vi "APDM Get Gyro Data.vi"(5 "Sim Gyro Cluster":T1, 8 "Gyro Data":T3={"Time"=0.0, "Normalization Time"=640.0, "Sampling Rate"=0.0, "Left Gyro Data"={"Time"=0.0, "Gyro Array Data"=[], "Gyro Negation"=[], "Gyro Data"={"Gyro X"=0.0, "Gyro Y"=0.0, "Gyro Z"=0.0}, "Gyro Latency"=0.0, "Normalization Time"=0.0, "Sampling Rate"=0.0}, "Right Gyro Data"={"Time"=0.0, "Gyro Array Data"=[], "Gyro Negation"=[], "Gyro Data"={"Gyro X"=0.0, "Gyro Y"=0.0, "Gyro Z"=0.0}, "Gyro Latency"=0.0, "Normalization Time"=0.0, "Sampling Rate"=0.0}}, 9 "APDM Context":T6={"APDM Context ID"=0, "Gyro Mode"="", "Log Data"=FALSE, "Log File"=refnum, "Gyro Record Log"=refnum, "Gyro CMD Log"=refnum, "L Opal SN"=0, "R Opal SN"=0, "Access Point ID"=0, "Left Gyro Sim Data"=path "C:/Users/jfalesi/Desktop/CP FES Walking Code/Original/Ahad Vi/CP Code/Offline data/TD_7_Raw_R.txt", "Right Gyro Sim Data"=path "C:/Users/jfalesi/Desktop/CP FES Walking Code/Original/Ahad Vi/CP Code/Offline data/TD_7_Raw_R.txt", "Sampling Rate"=0.0, "Gyro Sim Time Array"=[], "Missed Gyro Count"=0.0}) -> (1 "Cmd Log String":string, 2 "Gyro Data":T3={"Time"=0.0, "Normalization Time"=640.0, "Sampling Rate"=0.0, "Left Gyro Data"={"Time"=0.0, "Gyro Array Data"=[], "Gyro Negation"=[], "Gyro Data"={"Gyro X"=0.0, "Gyro Y"=0.0, "Gyro Z"=0.0}, "Gyro Latency"=0.0, "Normalization Time"=0.0, "Sampling Rate"=0.0}, "Right Gyro Data"={"Time"=0.0, "Gyro Array Data"=[], "Gyro Negation"=[], "Gyro Data"={"Gyro X"=0.0, "Gyro Y"=0.0, "Gyro Z"=0.0}, "Gyro Latency"=0.0, "Normalization Time"=0.0, "Sampling Rate"=0.0}}, 3 "APDM Context Out out":T6={"APDM Context ID"=0, "Gyro Mode"="", "Log Data"=FALSE, "Log File"=refnum, "Gyro Record Log"=refnum, "Gyro CMD Log"=refnum, "L Opal SN"=0, "R Opal SN"=0, "Access Point ID"=0, "Left Gyro Sim Data"=path "C:/Users/jfalesi/Desktop/CP FES Walking Code/Original/Ahad Vi/CP Code/Offline data/TD_7_Raw_R.txt", "Right Gyro Sim Data"=path "C:/Users/jfalesi/Desktop/CP FES Walking Code/Original/Ahad Vi/CP Code/Offline data/TD_7_Raw_R.txt", "Sampling Rate"=0.0, "Gyro Sim Time Array"=[], "Missed Gyro Count"=0.0}, 4 "Data Log Item":T2)   [LabVIEW 2019]
uses:
  Controls/APDM Context Cluster.ctl
  Controls/Gyro Data.ctl
  Controls/Gyro Side Data.ctl
  Controls/Gyro Negation.ctl
  Controls/Gyro Data Log Item.ctl
  Archive/CP_FES_Walking_w_stim_on_off.llb/Left_Right_Control.ctl
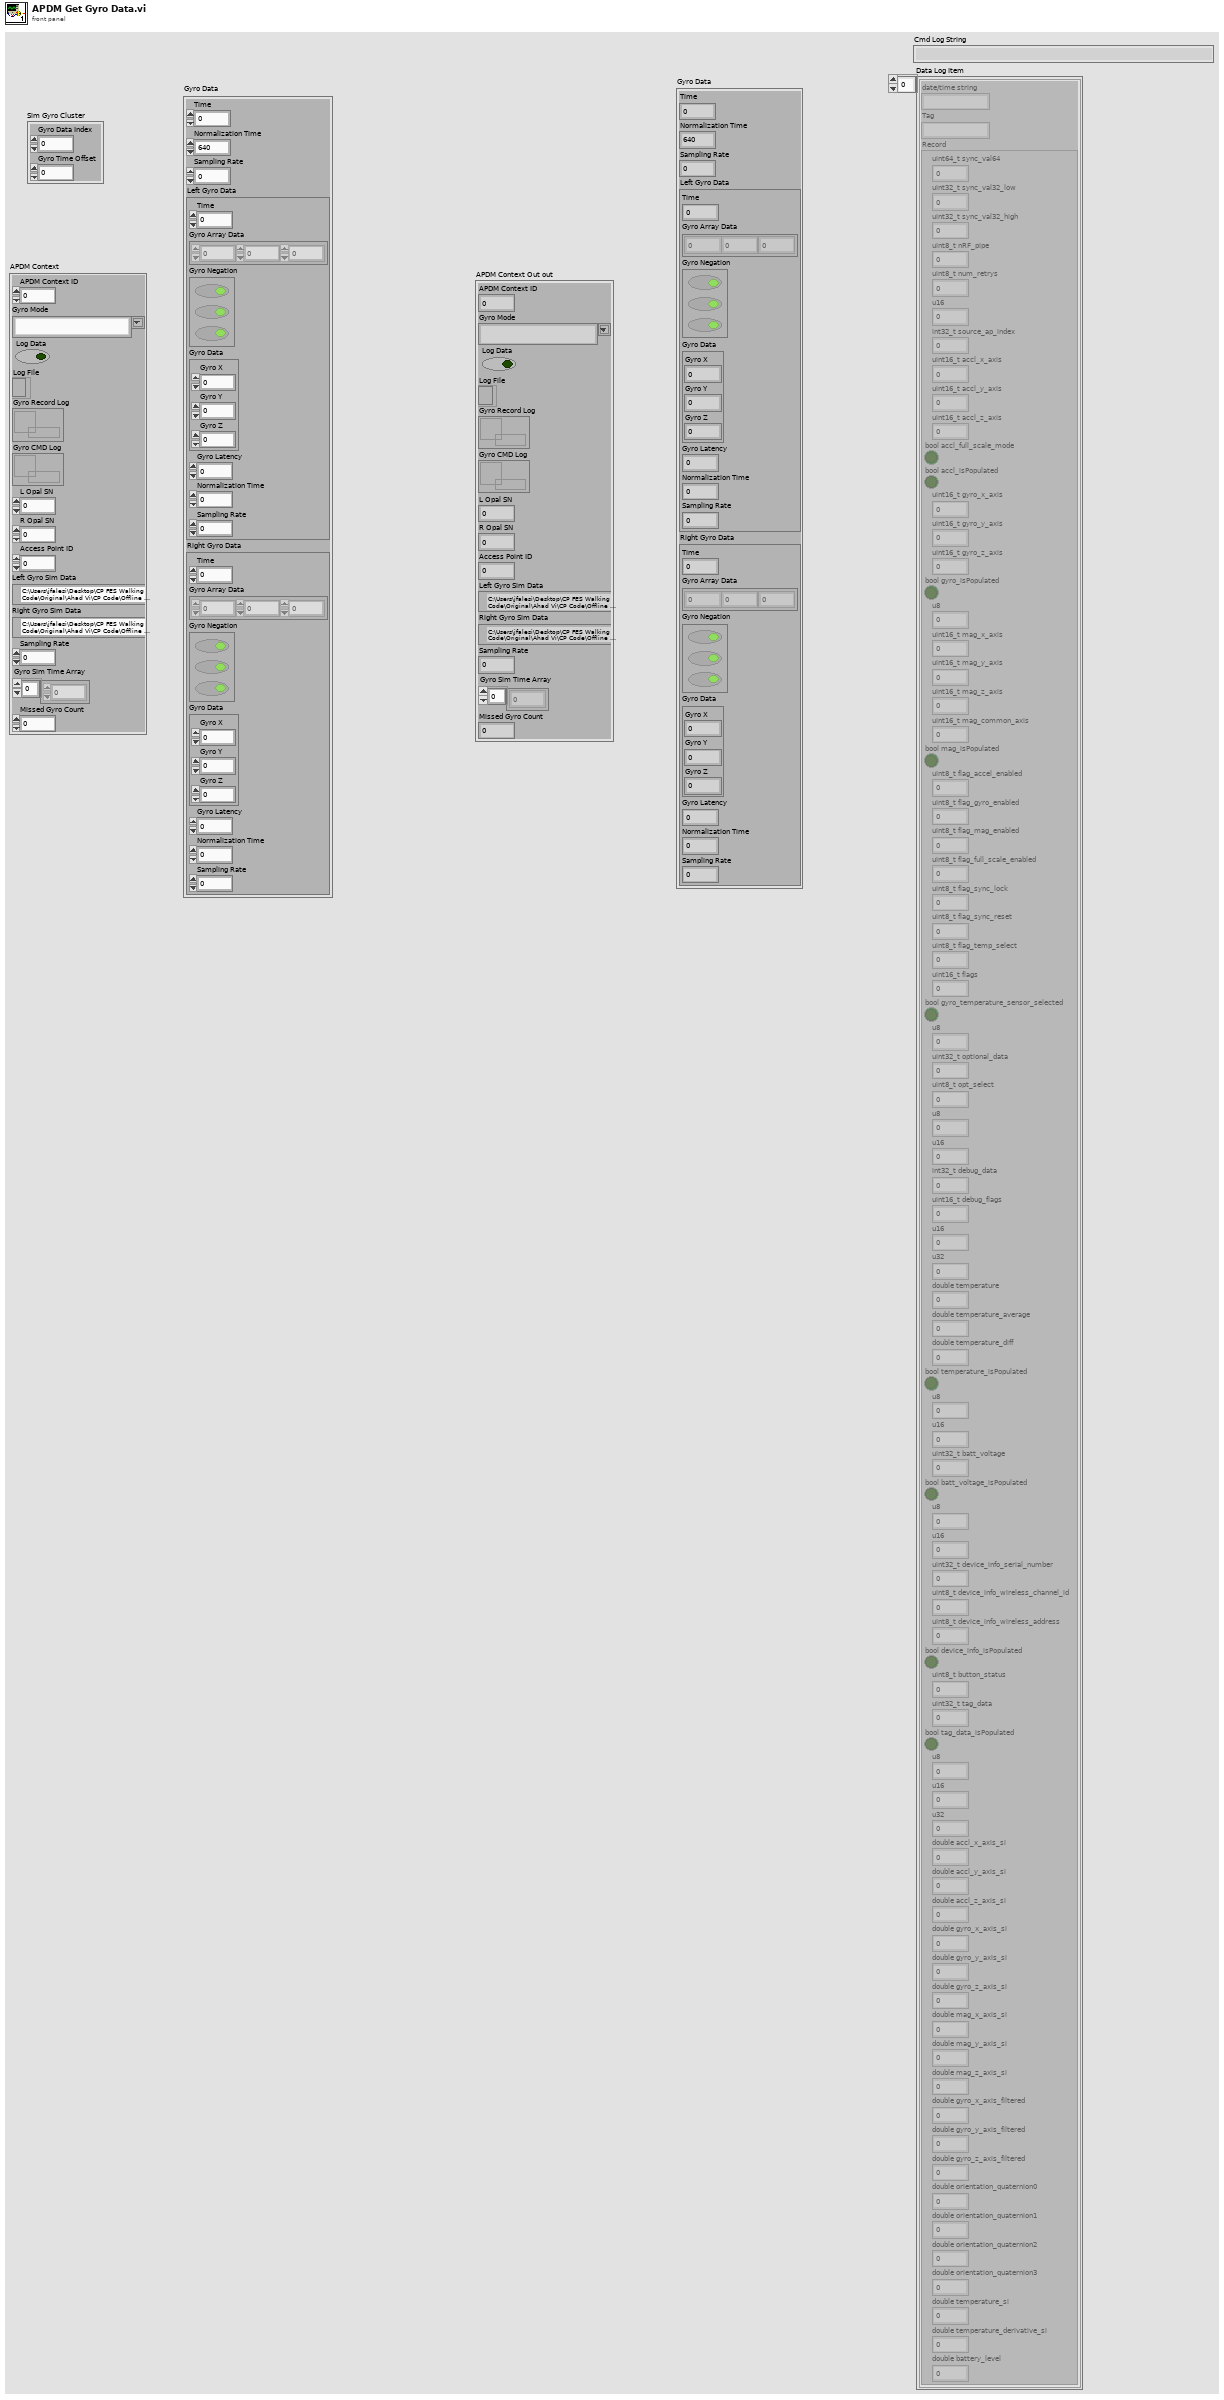
[diagram p1: front panel]
types:
  T1 = cluster{"Gyro Data Index":i32, "Gyro Time Offset":dbl}
  T2 = typedef "Gyro Data Log Item.ctl" = cluster{"date/time string":string, "Tag":string, "Record":cluster{"uint64_t sync_val64":u64, "uint32_t sync_val32_low":u32, "uint32_t sync_val32_high":u32, "uint8_t nRF_pipe":u8, "uint8_t num_retrys":u8, "u16":u16, "int32_t source_ap_index":i32, "uint16_t accl_x_axis":u16, "uint16_t accl_y_axis":u16, "uint16_t accl_z_axis":u16, "bool accl_full_scale_mode":bool, "bool accl_isPopulated":bool, "uint16_t gyro_x_axis":u16, "uint16_t gyro_y_axis":u16, "uint16_t gyro_z_axis":u16, "bool gyro_isPopulated":bool, "u8":u8, "uint16_t mag_x_axis":u16, "uint16_t mag_y_axis":u16, "uint16_t mag_z_axis":u16, "uint16_t mag_common_axis":u16, "bool mag_isPopulated":bool, "uint8_t flag_accel_enabled":u8, "uint8_t flag_gyro_enabled":u8, "uint8_t flag_mag_enabled":u8, "uint8_t flag_full_scale_enabled":u8, "uint8_t flag_sync_lock":u8, "uint8_t flag_sync_reset":u8, "uint8_t flag_temp_select":u8, "uint16_t flags":u16, "bool gyro_temperature_sensor_selected":bool, "u8":u8, "uint32_t optional_data":u32, "uint8_t opt_select":u8, "u8":u8, "u16":u16, "int32_t debug_data":i32, "uint16_t debug_flags":u16, "u16":u16, "u32":u32, "double temperature":dbl, "double temperature_average":dbl, "double temperature_diff":dbl, "bool temperature_isPopulated":bool, "u8":u8, "u16":u16, "uint32_t batt_voltage":u32, "bool batt_voltage_isPopulated":bool, "u8":u8, "u16":u16, "uint32_t device_info_serial_number":u32, "uint8_t device_info_wireless_channel_id":u8, "uint8_t device_info_wireless_address":u8, "bool device_info_isPopulated":bool, "uint8_t button_status":u8, "uint32_t tag_data":u32, "bool tag_data_isPopulated":bool, "u8":u8, "u16":u16, "u32":u32, "double accl_x_axis_si":dbl, "double accl_y_axis_si":dbl, "double accl_z_axis_si":dbl, "double gyro_x_axis_si":dbl, "double gyro_y_axis_si":dbl, "double gyro_z_axis_si":dbl, "double mag_x_axis_si":dbl, "double mag_y_axis_si":dbl, "double mag_z_axis_si":dbl, "double gyro_x_axis_filtered":dbl, "double gyro_y_axis_filtered":dbl, "double gyro_z_axis_filtered":dbl, "double orientation_quaternion0":dbl, "double orientation_quaternion1":dbl, "double orientation_quaternion2":dbl, "double orientation_quaternion3":dbl, "double temperature_si":dbl, "double temperature_derivative_si":dbl, "double battery_level":dbl}}[]
  T3 = typedef "Gyro Data.ctl" = cluster{"Time":dbl, "Normalization Time":dbl, "Sampling Rate":dbl, "Left Gyro Data":T4, "Right Gyro Data":T4}
  T4 = typedef "Gyro Side Data.ctl" = cluster{"Time":dbl, "Gyro Array Data":dbl[], "Gyro Negation":T5, "Gyro Data":cluster{"Gyro X":dbl, "Gyro Y":dbl, "Gyro Z":dbl}, "Gyro Latency":dbl, "Normalization Time":dbl, "Sampling Rate":dbl}
  T5 = typedef "Gyro Negation.ctl" = bool[]
  T6 = typedef "APDM Context Cluster.ctl" = cluster{"APDM Context ID":u32, "Gyro Mode":string, "Log Data":bool, "Log File":refnum<file>, "Gyro Record Log":refnum<queue>, "Gyro CMD Log":refnum<queue>, "L Opal SN":u32, "R Opal SN":u32, "Access Point ID":u32, "Left Gyro Sim Data":path, "Right Gyro Sim Data":path, "Sampling Rate":dbl, "Gyro Sim Time Array":dbl[], "Missed Gyro Count":dbl}
  T7 = typedef "Left_Right_Control.ctl" = string
  T8 = cluster{"date/time string":string, "Tag":string, "Record":cluster{"uint64_t sync_val64":u64, "uint32_t sync_val32_low":u32, "uint32_t sync_val32_high":u32, "uint8_t nRF_pipe":u8, "uint8_t num_retrys":u8, "u16":u16, "int32_t source_ap_index":i32, "uint16_t accl_x_axis":u16, "uint16_t accl_y_axis":u16, "uint16_t accl_z_axis":u16, "bool accl_full_scale_mode":bool, "bool accl_isPopulated":bool, "uint16_t gyro_x_axis":u16, "uint16_t gyro_y_axis":u16, "uint16_t gyro_z_axis":u16, "bool gyro_isPopulated":bool, "u8":u8, "uint16_t mag_x_axis":u16, "uint16_t mag_y_axis":u16, "uint16_t mag_z_axis":u16, "uint16_t mag_common_axis":u16, "bool mag_isPopulated":bool, "uint8_t flag_accel_enabled":u8, "uint8_t flag_gyro_enabled":u8, "uint8_t flag_mag_enabled":u8, "uint8_t flag_full_scale_enabled":u8, "uint8_t flag_sync_lock":u8, "uint8_t flag_sync_reset":u8, "uint8_t flag_temp_select":u8, "uint16_t flags":u16, "bool gyro_temperature_sensor_selected":bool, "u8":u8, "uint32_t optional_data":u32, "uint8_t opt_select":u8, "u8":u8, "u16":u16, "int32_t debug_data":i32, "uint16_t debug_flags":u16, "u16":u16, "u32":u32, "double temperature":dbl, "double temperature_average":dbl, "double temperature_diff":dbl, "bool temperature_isPopulated":bool, "u8":u8, "u16":u16, "uint32_t batt_voltage":u32, "bool batt_voltage_isPopulated":bool, "u8":u8, "u16":u16, "uint32_t device_info_serial_number":u32, "uint8_t device_info_wireless_channel_id":u8, "uint8_t device_info_wireless_address":u8, "bool device_info_isPopulated":bool, "uint8_t button_status":u8, "uint32_t tag_data":u32, "bool tag_data_isPopulated":bool, "u8":u8, "u16":u16, "u32":u32, "double accl_x_axis_si":dbl, "double accl_y_axis_si":dbl, "double accl_z_axis_si":dbl, "double gyro_x_axis_si":dbl, "double gyro_y_axis_si":dbl, "double gyro_z_axis_si":dbl, "double mag_x_axis_si":dbl, "double mag_y_axis_si":dbl, "double mag_z_axis_si":dbl, "double gyro_x_axis_filtered":dbl, "double gyro_y_axis_filtered":dbl, "double gyro_z_axis_filtered":dbl, "double orientation_quaternion0":dbl, "double orientation_quaternion1":dbl, "double orientation_quaternion2":dbl, "double orientation_quaternion3":dbl, "double temperature_si":dbl, "double temperature_derivative_si":dbl, "double battery_level":dbl}}
  T9 = typedef "Data From Gyro.ctl" = cluster{"Gyro X":dbl, "Gyro Y":dbl, "Gyro Z":dbl, "Gyro Time":dbl}
  T10 = cluster{"date/time string":string, "Tag":string, "Record":cluster{"uint64_t sync_val64":u64, "uint32_t sync_val32_low":u32, "uint32_t sync_val32_high":u32, "uint8_t nRF_pipe":u8, "uint8_t num_retrys":u8, "u16":u16, "int32_t source_ap_index":i32, "uint16_t accl_x_axis":u16, "uint16_t accl_y_axis":u16, "uint16_t accl_z_axis":u16, "bool accl_full_scale_mode":bool, "bool accl_isPopulated":bool, "uint16_t gyro_x_axis":u16, "uint16_t gyro_y_axis":u16, "uint16_t gyro_z_axis":u16, "bool gyro_isPopulated":bool, "u8":u8, "uint16_t mag_x_axis":u16, "uint16_t mag_y_axis":u16, "uint16_t mag_z_axis":u16, "uint16_t mag_common_axis":u16, "bool mag_isPopulated":bool, "uint8_t flag_accel_enabled":u8, "uint8_t flag_gyro_enabled":u8, "uint8_t flag_mag_enabled":u8, "uint8_t flag_full_scale_enabled":u8, "uint8_t flag_sync_lock":u8, "uint8_t flag_sync_reset":u8, "uint8_t flag_temp_select":u8, "uint16_t flags":u16, "bool gyro_temperature_sensor_selected":bool, "u8":u8, "uint32_t optional_data":u32, "uint8_t opt_select":u8, "u8":u8, "u16":u16, "int32_t debug_data":i32, "uint16_t debug_flags":u16, "u16":u16, "u32":u32, "double temperature":dbl, "double temperature_average":dbl, "double temperature_diff":dbl, "bool temperature_isPopulated":bool, "u8":u8, "u16":u16, "uint32_t batt_voltage":u32, "bool batt_voltage_isPopulated":bool, "u8":u8, "u16":u16, "uint32_t device_info_serial_number":u32, "uint8_t device_info_wireless_channel_id":u8, "uint8_t device_info_wireless_address":u8, "bool device_info_isPopulated":bool, "uint8_t button_status":u8, "uint32_t tag_data":u32, "bool tag_data_isPopulated":bool, "u8":u8, "u16":u16, "u32":u32, "double accl_x_axis_si":dbl, "double accl_y_axis_si":dbl, "double accl_z_axis_si":dbl, "double gyro_x_axis_si":dbl, "double gyro_y_axis_si":dbl, "double gyro_z_axis_si":dbl, "double mag_x_axis_si":dbl, "double mag_y_axis_si":dbl, "double mag_z_axis_si":dbl, "double gyro_x_axis_filtered":dbl, "double gyro_y_axis_filtered":dbl, "double gyro_z_axis_filtered":dbl, "double orientation_quaternion0":dbl, "double orientation_quaternion1":dbl, "double orientation_quaternion2":dbl, "double orientation_quaternion3":dbl, "double temperature_si":dbl, "double temperature_derivative_si":dbl, "double battery_level":dbl}}[]
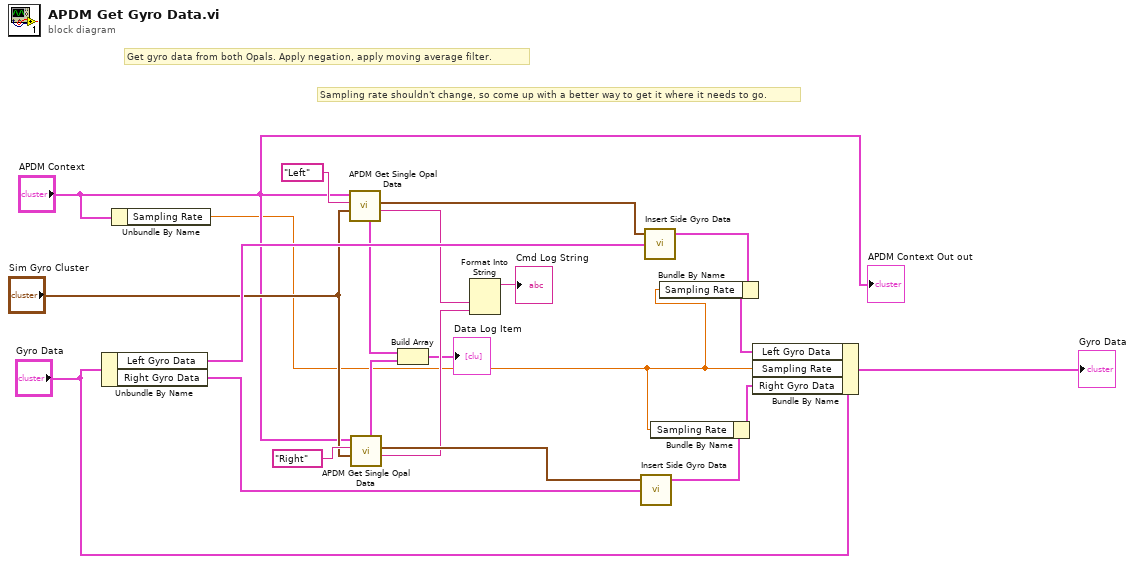
[diagram p0: block diagram]
diagram:
  # "Sampling rate shouldn't change, so come up with a better way to get it where it needs to go."
  # "Get gyro data from both Opals. Apply negation, apply moving average filter."
  n1 = Unbundle By Name("Gyro Data") -> ("Left Gyro Data"=w19:T4, "Right Gyro Data"=w15:T4)
  n2 = Unbundle By Name("APDM Context") -> ("Sampling Rate"=w1:dbl)
  n3 = call "APDM Get Single Opal Data.vi"("APDM Context"="APDM Context", "Left or Right"=T7 "Left", "Sim Gyro Cluster"="Sim Gyro Cluster") -> ("Data Log Item"=w5:T8, "Data from Gyro"=w13:T9, "Cmd Log String"=w9:string)  [unwired: 2 in, 1 out]
  n4 = call "APDM Get Single Opal Data.vi"("APDM Context"="APDM Context", "Left or Right"=T7 "Right", "Sim Gyro Cluster"="Sim Gyro Cluster") -> ("Data Log Item"=w6:T8, "Data from Gyro"=w14:T9, "Cmd Log String"=w8:string)  [unwired: 2 in, 1 out]
  n5 = Build Array(w5, w6) -> (→"Data Log Item":T10)
  n6 = Format Into String(w9, w8) -> (resulting string=→"Cmd Log String":string)  [unwired: 3 in, 1 out]
  n7 = call "Insert Side Gyro Data.vi"("Side Gyro Data in"=w15, "Data from Gyro"=w14) -> ("Side Gyro Data out"=w17:T4)  [unwired: 3 in]
  n8 = call "Insert Side Gyro Data.vi"("Side Gyro Data in"=w19, "Data from Gyro"=w13) -> ("Side Gyro Data out"=w11:T4)  [unwired: 3 in]
  n9 = Bundle By Name(cluster=w17, "Sampling Rate"=w1) -> (w12:T4)
  n10 = Bundle By Name(cluster=w11, "Sampling Rate"=w1) -> (w10:T4)
  n11 = Bundle By Name(cluster="Gyro Data", "Left Gyro Data"=w10, "Sampling Rate"=w1, "Right Gyro Data"=w12) -> (→"Gyro Data":T3)
  "APDM Context Out out" <- "APDM Context"
